vi "Matlab clear and close all.vi"(8 "error in (no error)":errorcluster) -> (0 "error out":errorcluster)   [LabVIEW 2013]
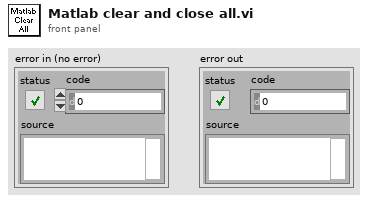
[diagram p1: front panel]
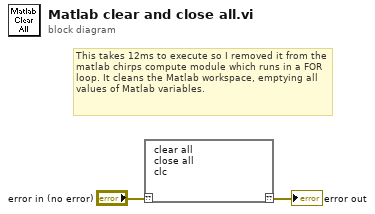
[diagram p0: block diagram]
diagram:
  # "This takes 12ms to execute so I removed it from the matlab chirps compute module which runs in a FOR loop. It cleans the Matlab workspace, emptying all values of Matlab variables."
  n1 = script code="clear all\nclose all\nclc" ("Script Node")("??"="error in (no error)") -> ("??"=→"error out":errorcluster)
